vi "Unflatten.vi"(8 "error in":errorcluster, 10 "Buffer":u8[](array[numeric]) format="%.0x") -> (0 "error out":errorcluster, 2 "Command Data":T1 {"Time Stamp" format="%<%x %.3X>T"})   [LabVIEW 2023, in "ConstellationCommand.lvlib"]
uses:
  <vilib>/IlluminatedG/IG Protoc/LV-Proto/Wire Decode Varint I32.vi
  <vilib>/IlluminatedG/IG Protoc/LV-Proto/Extract Varint Bytes.vi
  ConstellationCommand.lvlib
  <vilib>/IlluminatedG/IG Protoc/LV-Proto/LV-Proto.lvlib
  Data.ctl
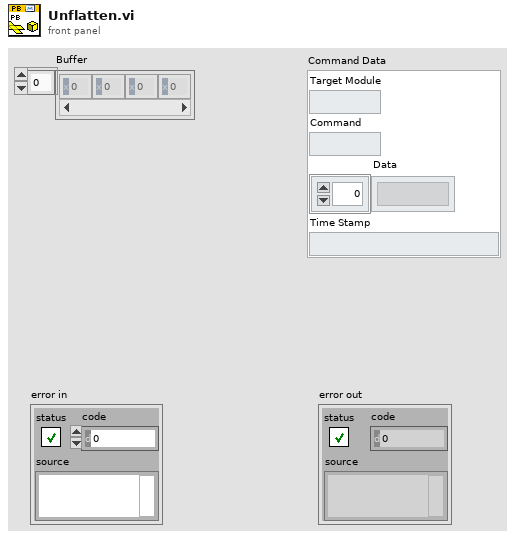
[diagram p1: front panel]
types:
  T1 = typedef "ConstellationCommand.lvlib/Data.ctl" = cluster{"Target Module":string, "Command":string, "Data":string[], "Time Stamp":timestamp}
  T2 = typedef "LV-Proto.lvlib/Wire Type.ctl" = enum8{"VARINT", "I64", "LEN", "SGROUP (Deprecated)", "EGROUP (Deprecated)", "I32"}
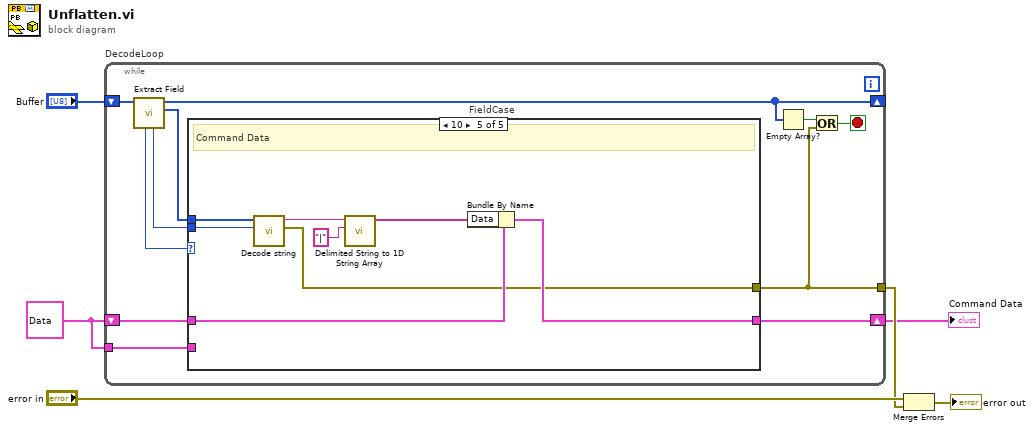
[diagram p0: block diagram]
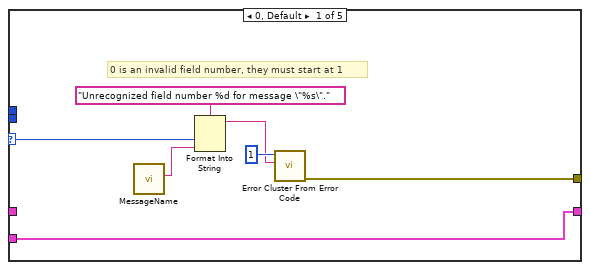
[diagram p2: hidden frame]
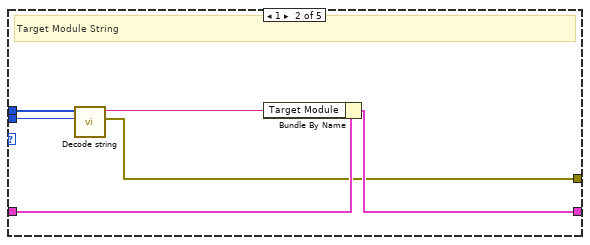
[diagram p3: hidden frame]
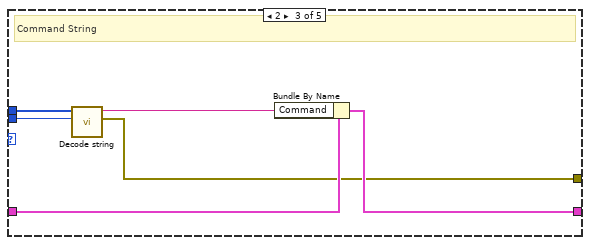
[diagram p4: hidden frame]
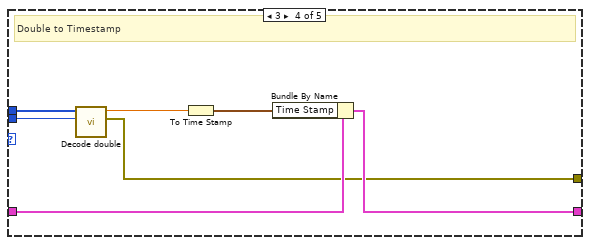
[diagram p5: hidden frame]
diagram:
  w2 = T1 {"Target Module"="", "Command"="", "Data"=[], "Time Stamp"=timestamp(0 s since 1904-01-01)} ("Command Data")
  n1 = while "DecodeLoop" {
    shift-right: [w16] -> _
    shift-left: "Buffer" -> [w17]
    shift-right: [w9] -> w1
    shift-left: w2 -> [w15]
    tunnel: [w8] -> w4
    tunnel: w2 -> [w7]
    stop <- w11 stop-if-true
    n2 = call <vilib>:"Extract Field.vi"("Buffer in"=w17) -> ("Field Data"=w10:u8[], "Buffer"=w16:u8[], "Wire Type"=w13:T2, "Field Number"=w14:i32)  [unwired: 7 in]
    n3 = case "FieldCase" shown="10" w14 {
      selector: w14 -> [w23 _ _ _ _]
      tunnel: w15 -> [_ w30 w36 w43 w51]
      tunnel: w13 -> [_ w27 w33 w40 w48]
      tunnel: w10 -> [_ w28 w34 w41 w49]
      tunnel: [w19 w29 w35 w42 w50] -> w9
      tunnel: [w20 w25 w31 w39 w44] -> w8
      tunnel: w7 -> [w19 _ _ _ _]
      frame 0, Default {
        # "0 is an invalid field number, they must start at 1"
        n4 = call "MessageName.vi"() -> ("MessageName"=w18:string)  [unwired: 11 in]
        n5 = Format Into String(format string="Unrecognized field number %d for message \"%s\".", w23, w18) -> (resulting string=w21:string)  [unwired: 2 in, 1 out]
        n6 = call <vilib>:"Error Cluster From Error Code.vi"("error message (\"\")"=w21, "error code (0)"=1) -> ("error out"=w20:errorcluster)  [unwired: 7 in]
      }
      frame 1 {
        # "Target Module String"
        n7 = call <vilib>:"Decode string.vi"("Wire Type"=w27, "Data"=w28) -> ("error out"=w25:errorcluster, "string"=w26:string)  [unwired: 8 in]
        n8 = Bundle By Name(cluster=w30, "Target Module"=w26) -> (w29:T1)
      }
      frame 2 {
        # "Command String"
        n9 = call <vilib>:"Decode string.vi"("Wire Type"=w33, "Data"=w34) -> ("error out"=w31:errorcluster, "string"=w32:string)  [unwired: 8 in]
        n10 = Bundle By Name(cluster=w36, "Command"=w32) -> (w35:T1)
      }
      frame 3 {
        # "Double to Timestamp"
        n11 = call <vilib>:"Decode double.vi"("Wire Type"=w40, "Data"=w41) -> ("error out"=w39:errorcluster, "double"=w38:dbl)  [unwired: 8 in]
        n12 = To Time Stamp(1:w38) -> (0:w37:timestamp)
        n13 = Bundle By Name(cluster=w43, "Time Stamp"=w37) -> (w42:T1)
      }
      frame 10 {
        # "Command Data"
        n14 = call <vilib>:"Decode string.vi"("Wire Type"=w48, "Data"=w49) -> ("error out"=w44:errorcluster, "string"=w47:string)  [unwired: 8 in]
        n15 = call <vilib>:"Delimited String to 1D String Array.vi"("delimiter"="|", "delimited string"=w47) -> ("string array"=w46:string[])  [unwired: 9 in]
        n16 = Bundle By Name(cluster=w51, "Data"=w46) -> (w50:T1)
      }
    }
    n17 = Empty Array?(array=w16) -> (empty?=w12:bool)
    n18 = Or(x=w12, y=w8) -> (x .or. y?=w11:bool)
  }
  "Command Data" <- w1
  n19 = Merge Errors("error in", w4) -> (→"error out":errorcluster)
